vi "myRIO_BRig_Host_testRandomize.vi"() -> ()   [LabVIEW 2014]
panel:
  out "Waveform Chart":u16[](graph)
  in  "stop":bool
  out "x/y":dbl
  in  "Numeric":u16
  in  "Input_Min":u16=1 min=1 step=1
  in  "Input_Max":u16=1 min=1 step=1
  in  "Input_Increment":u16=1 step=1
  out "Output":u16
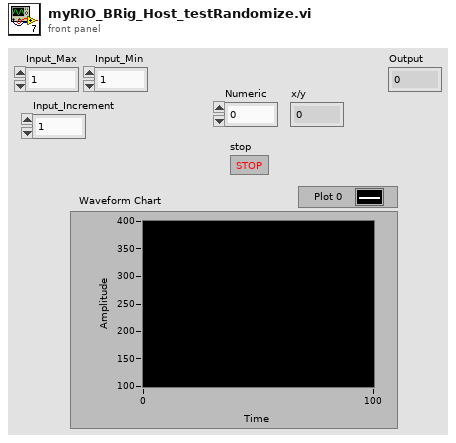
[diagram p1: front panel]
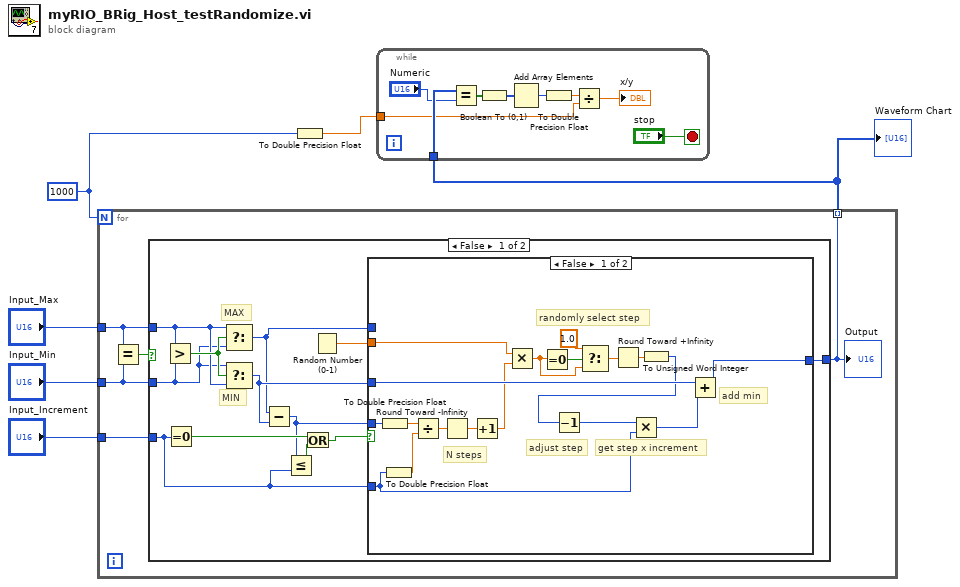
[diagram p0: block diagram]
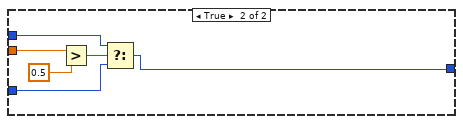
[diagram p2: hidden frame]
diagram:
  w3 = 1000
  n1 = for {
    N: w3 -> [_]
    tunnel: "Input_Max" -> [w10]
    tunnel: "Input_Min" -> [w9]
    tunnel: "Input_Increment" -> [w8]
    tunnel: [w7] -> w1 mode=indexing
    n2 = Equal?(x=w10, y=w9) -> (x = y?=w11:bool)
    n3 = case shown="False" w11 {
      tunnel: w10 -> [w21 w48]
      tunnel: w9 -> [w20 _]
      tunnel: [w23 w48] -> w7
      tunnel: w8 -> [w17 _]
      frame False {
        # "MIN"
        # "MAX"
        n4 = Greater?(x=w21, y=w20) -> (0:w22:bool)
        n5 = Equal To 0?(x=w17) -> (x = 0?=w15:bool)
        n6 = Select(t=w21, s=w22, f=w20) -> (s? t:f=w18:u16)
        n7 = Select(t=w20, s=w22, f=w21) -> (s? t:f=w19:u16)
        n8 = Subtract(x=w18, y=w19) -> (x-y=w12:u16)
        n9 = Less Or Equal?(x=w12, y=w17) -> (x <= y?=w16:bool)
        n10 = Or(x=w15, y=w16) -> (x .or. y?=w14:bool)
        n11 = Random Number (0-1)() -> (number: 0 to 1=w13:dbl)
        n12 = case shown="False" w14 {
          tunnel: w18 -> [_ w45]
          tunnel: w19 -> [w33 w44]
          tunnel: [w32 w43] -> w23
          tunnel: w17 -> [w35 _]
          tunnel: w13 -> [w37 w42]
          tunnel: w12 -> [w41 _]
          frame False {
            # "add min"
            # "get step x increment"
            # "adjust step"
            # "randomly select step"
            # "N steps"
            n13 = To Double Precision Float(number=w41) -> (double precision float=w40:dbl)
            n14 = To Double Precision Float(number=w35) -> (double precision float=w39:dbl)
            n15 = Divide(x=w40, y=w39) -> (x/y=w38:dbl)
            n16 = Round Toward -Infinity(1:w38) -> (0:w31:dbl)
            n17 = Increment(x=w31) -> (x+1=w30:dbl)
            n18 = Multiply(x=w37, y=w30) -> (x*y=w28:dbl)
            n19 = Equal To 0?(x=w28) -> (x = 0?=w29:bool)
            n20 = Select(t=1.0, s=w29, f=w28) -> (s? t:f=w26:dbl)
            n21 = Round Toward +Infinity(x=w26) -> (ceil(x): smallest int >= x=w36:dbl)
            n22 = To Unsigned Word Integer(number=w36) -> (unsigned 16bit integer=w25:u16)
            n23 = Decrement(x=w25) -> (x-1=w24:u16)
            n24 = Multiply(x=w24, y=w35) -> (x*y=w34:u16)
            n25 = Add(x=w33, y=w34) -> (x+y=w32:u16)
          }
          frame True {
            n26 = Greater?(x=w42, y=0.5) -> (0:w46:bool)
            n27 = Select(t=w45, s=w46, f=w44) -> (s? t:f=w43:u16)
          }
        }
      }
      frame True {
      }
    }
    "Output" <- w7
  }
  "Waveform Chart" <- w1
  n28 = To Double Precision Float(number=w3) -> (double precision float=w2:dbl)
  n29 = while {
    tunnel: w1 -> [w57]
    tunnel: w2 -> [w52]
    stop <- "stop" stop-if-true
    n30 = Equal?(x=w57, y="Numeric") -> (x = y?=w56:bool[])
    n31 = Boolean To (0,1)(Boolean=w56) -> (0, 1=w55:i16[])
    n32 = Add Array Elements(numeric array=w55) -> (sum=w54:i16)
    n33 = To Double Precision Float(number=w54) -> (double precision float=w53:dbl)
    n34 = Divide(x=w53, y=w52) -> (x/y=→"x/y":dbl)
  }
